vi "k.vi"(8 "zeta":dbl=0.7, 9 "b":dbl=2.0, 10 "omega_d":dbl, 11 "v_d":dbl) -> (3 "k":dbl)   [LabVIEW 2023]
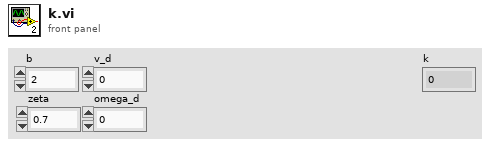
[diagram p1: front panel]
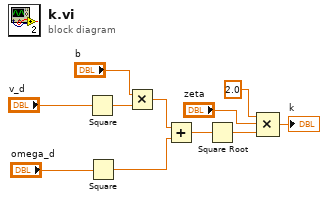
[diagram p0: block diagram]
diagram:
  n1 = Square(x="v_d") -> (x^2=w9:dbl)
  n2 = Square(x="omega_d") -> (x^2=w6:dbl)
  n3 = Multiply(x="b", y=w9) -> (x*y=w7:dbl)
  n4 = Add(x=w7, y=w6) -> (x+y=w5:dbl)
  n5 = Square Root(x=w5) -> (sqrt(x)=w4:dbl)
  n6 = Compound Arithmetic op=MULTIPLY(2.0 ("value"), "zeta", w4) -> (→"k":dbl)
